vi "Output Waveform Simulator.vi"() -> ()   [LabVIEW 2024]
uses:
  Waform generation/I-V parameters.ctl
  RP I-V Configuration.ctl
  Waform generation/Waveform parameters.ctl
panel:
  out "Waveform parameters out":T1={"Start magnitude"=1000.0, "Magnitude increment"=500.0, "Number of pulses"=8, "Ramp length"=32, "Top  length"=480, "Threshold "=15729, "Processing delay"=240, "Stop after"=480, "Detector window"=480, "Upper limit"=8191, "Lower limit"=-8192} {"Lower limit" format="%d (0x%x)"; "Upper limit" format="%d (0x%x)"; "Detector window" format="%dpts"; "Stop after" format="%d sweep(s)"}
  out "Output Waveform":dbl[][](graph)
  in  "Configuration":T2={"I-V parameters"={"Start magnitude"=0.001, "Magnitude increment"=0.001, "End magnitude"=0.01, "Ramp length"=32, "Top  length"=480, "Threshold "=0.0001, "Processing delay"=22, "Output gain "=480.0, "Interpolation"=64, "Stop after"=0, "Detector window"=480}, "Ranges"=[1.0, 1.0], "Post-trigger delay"=0.01, "Post-trigger duration"=0.1, "Output delay"=0.1, "Re-name chans"=["V", "I", "Vavg", "Pnum"]} {"Output delay" format="%#_6ps"; "Post-trigger duration" format="%#_6ps"; "Post-trigger delay" format="%#_6ps"; "Ranges" format="%#_6pV"; "I-V parameters"."Detector window" format="%dpts"; "I-V parameters"."Stop after" format="%d sweep(s)"; "I-V parameters"."Output gain" format="%#_6pA/V"; "I-V parameters"."Processing delay" format="%dpts"; "I-V parameters"."Threshold" format="%#_6pV"; "I-V parameters"."Top  length" format="%dpts"; "I-V parameters"."Ramp length" format="%dpts"; "I-V parameters"."End magnitude" format="%#_6pA"; "I-V parameters"."Magnitude increment" format="%#_6pA"; "I-V parameters"."Start magnitude" format="%#_6pA"}
  # "Waveform parameters"
  # "Detector parameters"
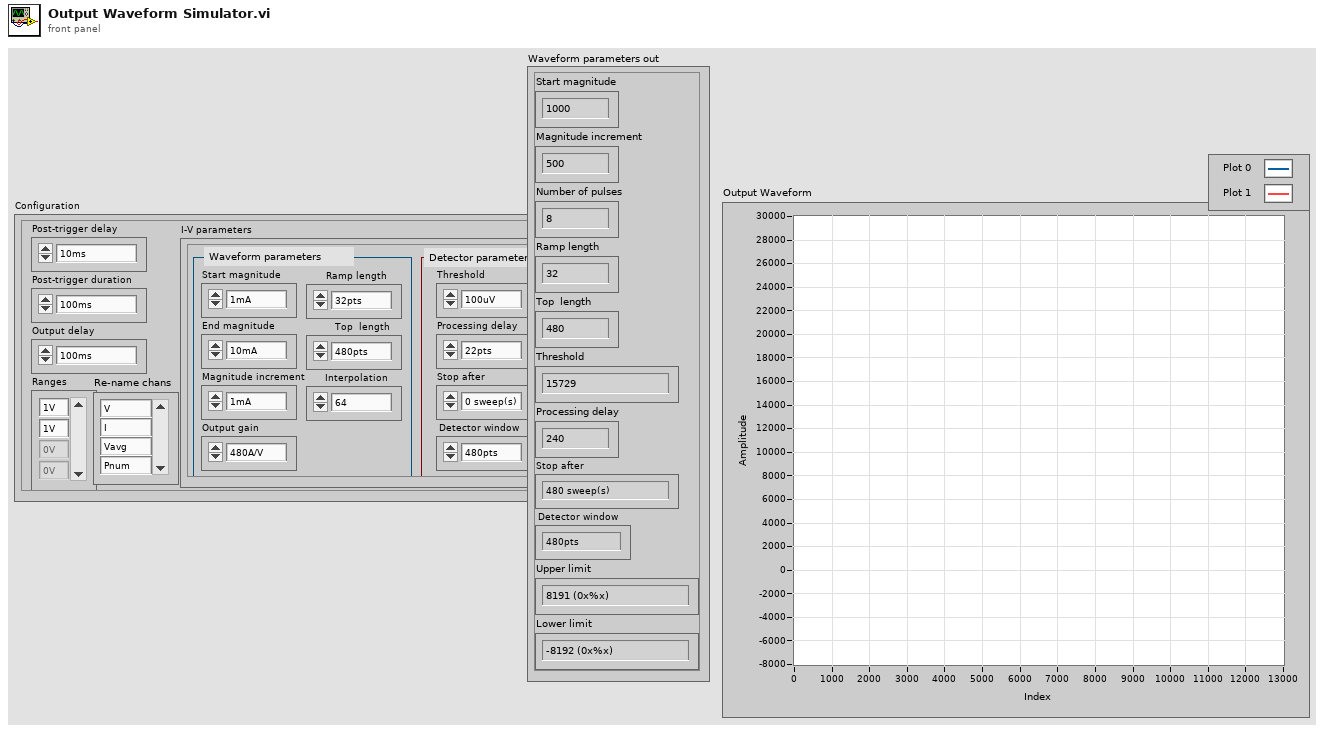
[diagram p1: front panel]
types:
  T1 = typedef "Waveform parameters.ctl" = cluster{"Start magnitude":dbl, "Magnitude increment":dbl, "Number of pulses":i32, "Ramp length":i32, "Top  length":i32, "Threshold ":i32, "Processing delay":u16, "Stop after":u16, "Detector window":i32, "Upper limit":i16, "Lower limit":i16}
  T2 = typedef "RP I-V Configuration.ctl" = cluster{"I-V parameters":T3, "Ranges":dbl[], "Post-trigger delay":dbl, "Post-trigger duration":dbl, "Output delay":dbl, "Re-name chans":string[]}
  T3 = typedef "I-V parameters.ctl" = cluster{"Start magnitude":dbl, "Magnitude increment":dbl, "End magnitude":dbl, "Ramp length":i32, "Top  length":i32, "Threshold ":dbl, "Processing delay":u16, "Output gain ":dbl, "Interpolation":i32, "Stop after":u16, "Detector window":i32}
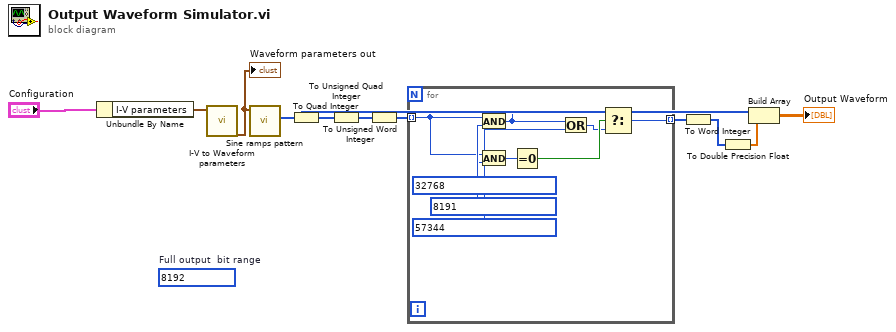
[diagram p0: block diagram]
diagram:
  (unwired) 8192  # Full output  bit range
  n1 = Unbundle By Name("Configuration") -> ("I-V parameters"=w10:T3)
  n2 = call "I-V to Waveform parameters.vi"("I-V parameters"=w10) -> ("Waveform parameters out"=w9:T1)  [unwired: 10 in]
  "Waveform parameters out" <- w9
  n3 = call "Sine ramps pattern.vi"("Waveform parameters 2"=w9) -> ("Waveform"=w8:i16[])  [unwired: 7 in, 2 out]
  n4 = To Quad Integer(1:w8) -> (0:w7:i64[])
  n5 = To Unsigned Quad Integer(1:w7) -> (0:w6:u64[])
  n6 = To Unsigned Word Integer(number=w6) -> (unsigned 16bit integer=w5:u16[])
  n7 = for {
    tunnel: w5 -> [w19] mode=indexing
    tunnel: [w15] -> w4 mode=indexing
    n8 = And(x=w19, y=u16 8191) -> (x .and. y?=w14:u16)
    n9 = And(x=w19, y=u16 32768) -> (x .and. y?=w17:u16)
    n10 = Equal To 0?(x=w17) -> (x = 0?=w16:bool)
    n11 = Or(x=w14, y=u16 57344) -> (x .or. y?=w12:u16)
    n12 = Select(t=w14, s=w16, f=w12) -> (s? t:f=w15:u16)
  }
  n13 = To Word Integer(number=w4) -> (16bit integer=w3:i16[])
  n14 = To Double Precision Float(number=w3) -> (double precision float=w1:dbl[])
  n15 = Build Array(w8, w1) -> (→"Output Waveform":dbl[][])
